vi "MotionCheck.vi"(8 "error in (no error)":errorcluster, 9 "In Motion?":refnum<vi>, 10 "UI":T1, 11 "CmdLib In":refnum<k24>) -> (0 "error out":errorcluster, 3 "CmdLib Out":refnum<k24>)   [LabVIEW 2022 SP3]
uses:
  C:/Development/rimas/RIMAS/Focus/PicoMotor/CmdLib.dll
  CmdLib.dll
  Global Variables.vi
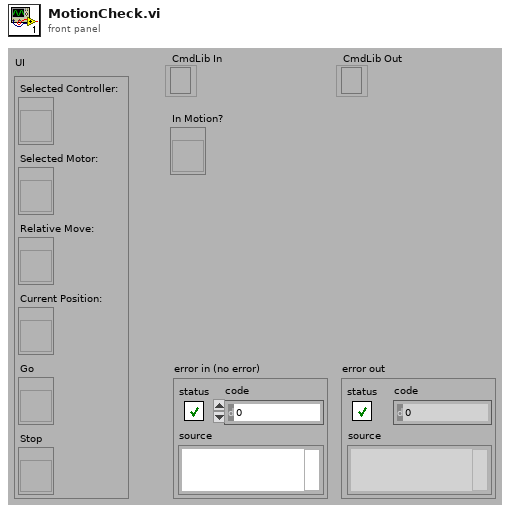
[diagram p1: front panel]
types:
  T1 = cluster{"Selected Controller:":refnum<vi>, "Selected Motor:":refnum<vi>, "Relative Move:":refnum<vi>, "Current Position:":refnum<vi>, "Go":refnum<vi>, "Stop":refnum<vi>}
  T2 = enum8{"Enabled", "Disabled", "Disabled and Grayed Out"}
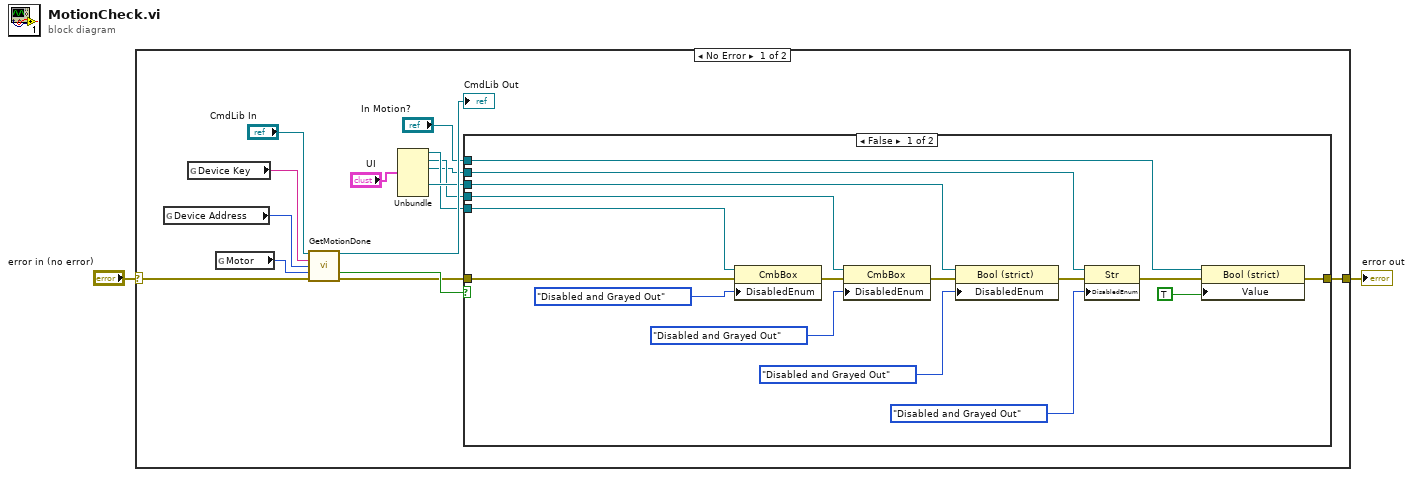
[diagram p0: block diagram]
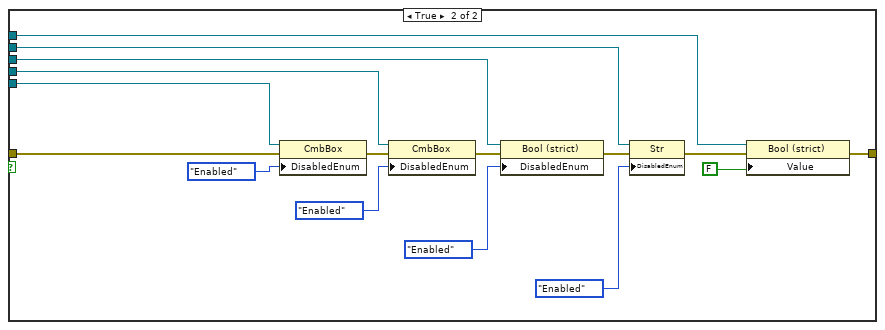
[diagram p2: hidden frame]
diagram:
  n1 = case shown="No Error" "error in (no error)" {
    selector: "error in (no error)" -> [w12 w50]
    tunnel: [w10 w50] -> w1
    frame No Error {
      n2 = global read "Global Variables.vi" "Device Address"() -> (w15:i32)
      n3 = global read "Global Variables.vi" "Device Key"() -> (w16:string)
      n4 = global read "Global Variables.vi" "Motor"() -> (w14:i32)
      n5 = call "GetMotionDone.vi"("CmdLib In"="CmdLib In", "DeviceKey In"=w16, "Device Address In"=w15, "Motor"=w14, "error in (no error)"=w12) -> ("CmdLib Out"=→"CmdLib Out":refnum<k24>, "Is Motion Done"=w13:bool, "error out"=w11:errorcluster)  [unwired: 6 in, 2 out]
      n6 = Unbundle("UI") -> ("Selected Controller:"=w5:refnum<vi>, "Selected Motor:"=w4:refnum<vi>, "Relative Move:"=w3:refnum<vi>, "Go"=w6:refnum<vi>)  [unwired: 2 out]
      n7 = case shown="False" w13 {
        tunnel: w6 -> [w32 w49]
        tunnel: w11 -> [w18 w43]
        tunnel: w3 -> [w31 w46]
        tunnel: [w19 w35] -> w10
        tunnel: w5 -> [w28 w41]
        tunnel: w4 -> [w26 w40]
        tunnel: "In Motion?" -> [w21 w37]
        frame False {
          n8 = property class="CmbBox"(reference=w28, error in=w18, "DisabledEnum"=T2."Disabled and Grayed Out" ("Disabled")) -> (error out=w23:errorcluster)  [unwired: 1 out]
          n9 = property class="CmbBox"(reference=w26, error in=w23, "DisabledEnum"=T2."Disabled and Grayed Out" ("Disabled")) -> (error out=w24:errorcluster)  [unwired: 1 out]
          n10 = property class="Bool (strict)"(reference=w32, error in=w24, "DisabledEnum"=T2."Disabled and Grayed Out" ("Disabled")) -> (error out=w33:errorcluster)  [unwired: 1 out]
          n11 = property class="Str"(reference=w31, error in=w33, "DisabledEnum"=T2."Disabled and Grayed Out" ("Disabled")) -> (error out=w20:errorcluster)  [unwired: 1 out]
          n12 = property class="Bool (strict)"(reference=w21, error in=w20, "Value"=TRUE) -> (error out=w19:errorcluster)  [unwired: 1 out]
        }
        frame True {
          n13 = property class="CmbBox"(reference=w41, error in=w43, "DisabledEnum"=T2."Enabled" ("Disabled")) -> (error out=w44:errorcluster)  [unwired: 1 out]
          n14 = property class="CmbBox"(reference=w40, error in=w44, "DisabledEnum"=T2."Enabled" ("Disabled")) -> (error out=w42:errorcluster)  [unwired: 1 out]
          n15 = property class="Bool (strict)"(reference=w49, error in=w42, "DisabledEnum"=T2."Enabled" ("Disabled")) -> (error out=w47:errorcluster)  [unwired: 1 out]
          n16 = property class="Str"(reference=w46, error in=w47, "DisabledEnum"=T2."Enabled" ("Disabled")) -> (error out=w34:errorcluster)  [unwired: 1 out]
          n17 = property class="Bool (strict)"(reference=w37, error in=w34, "Value"=FALSE) -> (error out=w35:errorcluster)  [unwired: 1 out]
        }
      }
    }
    frame Error {
    }
  }
  "error out" <- w1
